vi "UTIL_OpenFileDialog.vi"(10 "Root Name":string="PWC-OLS", 11 "relative path":path=path "$ReportFiles") -> (0 "selected path":path, 1 "File Name":string, 2 "Root Path":path)   [LabVIEW 2024]
doc: "Use to create relative paths to make the program portable.I\n\niNPUTS\nRelative Path is the name of the folder where to begin the file open dialog.\nRoot Name is the String name of the Root folder of this program.\n\nOUTPUS\nFile Path Path to the Opened File\nRoot Path Path to the root Folder\nFile Name String name less Path and extension."
uses:
  <vilib>/regexp/Match Regular Expression.xnode
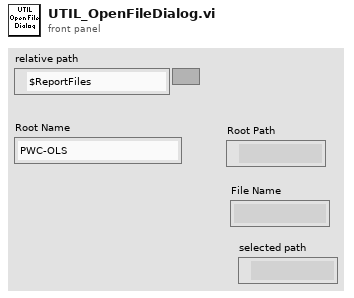
[diagram p1: front panel]
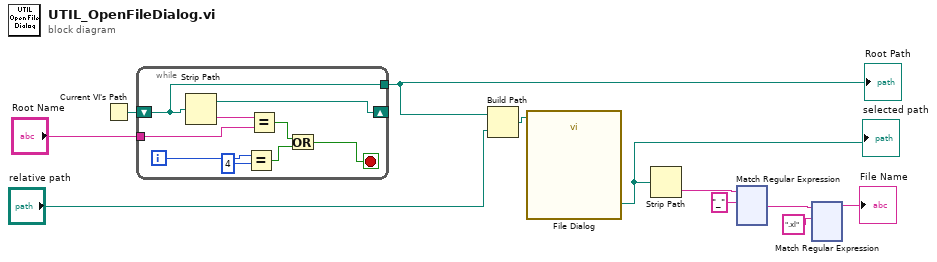
[diagram p0: block diagram]
diagram:
  n1 = Current VI's Path() -> (path=w11:path)
  n2 = while {
    shift-right: [w14] -> _
    shift-left: w11 -> [w13]
    tunnel: [w13] -> w8
    tunnel: "Root Name" -> [w12]
    i -> [w19]
    stop <- w15 stop-if-true
    n3 = Strip Path(path=w13) -> (stripped path=w14:path, name=w20:string)
    n4 = Equal?(x=w19, y=4) -> (x = y?=w16:bool)
    n5 = Equal?(x=w20, y=w12) -> (x = y?=w17:bool)
    n6 = Or(x=w17, y=w16) -> (x .or. y?=w15:bool)
  }
  "Root Path" <- w8
  n7 = Build Path(base path=w8, name or relative path="relative path") -> (appended path=w9:path)
  n8 = call "File Dialog"("start path"=w9) -> ("selected path"=w7:path)  [unwired: 11 in, 3 out]
  "selected path" <- w7
  n9 = Strip Path(path=w7) -> (name=w3:string)  [unwired: 1 out]
  n10 = xnode "Match Regular Expression"("input string"=w3, "regular expression"="_") -> ("after match"=w2:string)  [unwired: 4 in, 4 out]
  n11 = xnode "Match Regular Expression"("input string"=w2, "regular expression"=".xl") -> ("before match"=→"File Name":string)  [unwired: 4 in, 4 out]
